vi "Database.vi"() -> ()   [LabVIEW 2016]
uses:
  Database.Data.ctl
  Database.Data.Sets.ctl
  Handler/Database.Handler.Data.Status.ctl
  Database.Action.ctl
  Tools/CitTemplate/citTemplate.errData.ctl
  Tools/EventLog/EventLog.EventSource.ctl
  Database.Global.vi
panel:
  out "error.action":string
  out "error":errorcluster
  out "_loop":i32(ring)=4
  out "action":T1=enum."--- DB ---"
  out "Data":T2
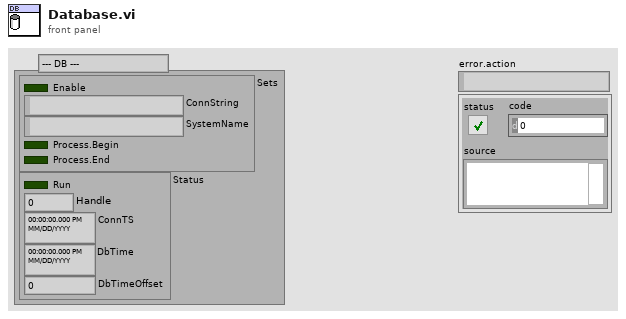
[diagram p1: front panel]
types:
  T1 = typedef "Database.Action.ctl" = enum32{"idle", "constructor", "destructor", "--- DB ---", "Setup", "Disconnect", "Connect", "GetAllStatuses"}
  T2 = typedef "Database.Data.ctl" = cluster{"Sets":T3, "Status":T4}
  T3 = typedef "Database.Data.Sets.ctl" = cluster{"Enable":bool, "ConnString":string, "SystemName":string, "Process.Begin":bool, "Process.End":bool}
  T4 = typedef "Database.Handler.Data.Status.ctl" = cluster{"Run":bool, "Handle":i32, "ConnTS":timestamp, "DbTime":timestamp, "DbTimeOffset":dbl}
  T5 = typedef "citTemplate.errData.ctl" = cluster{"ts":timestamp, "src":T6, "instance":i32, "action":string, "error":errorcluster, "unconfirmed":bool}
  T6 = typedef "EventLog.EventSource.ctl" = enum16{"All", "Gui", "Cache", "PLC1", "PLC2", "PLC3", "DB", "DB01", "DB02", "DB03", "DB04", "DB05", "DB06", "DB07", "DB08", "DB09", "DB10", "DB11", "DB12", "DB13", "DB14", "DB15", "DB16"}
  T7 = typedef "citTemplate.notifierHandle.ctl" = refnum<notifier>
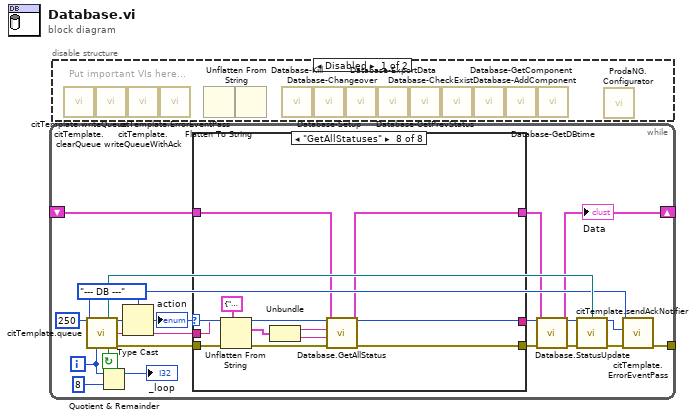
[diagram p0: block diagram]
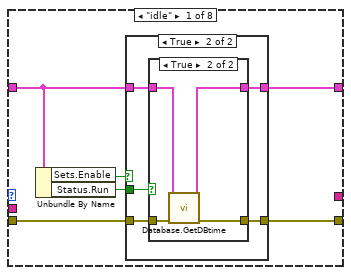
[diagram p3: hidden frame]
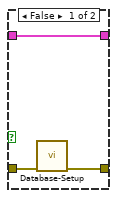
[diagram p5: hidden frame]
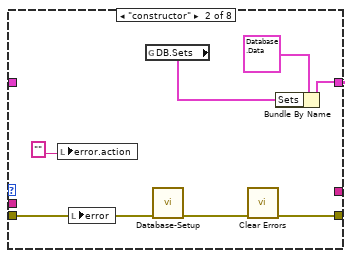
[diagram p6: hidden frame]
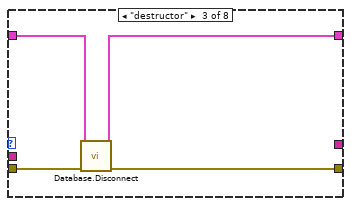
[diagram p7: hidden frame]
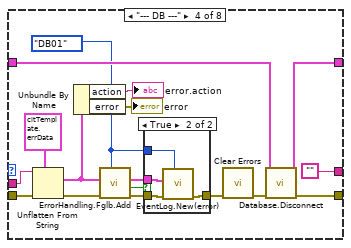
[diagram p8: hidden frame]
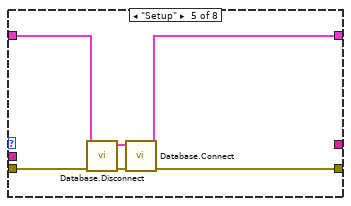
[diagram p10: hidden frame]
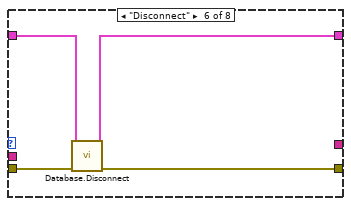
[diagram p11: hidden frame]
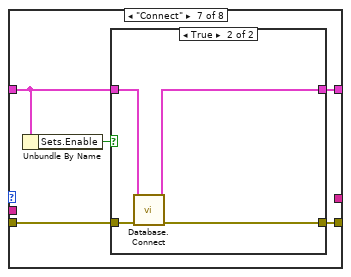
[diagram p12: hidden frame]
diagram:
  n1 = while {
    tunnel: [w12] -> _
    shift-right: [w1] -> _
    shift-left: _ -> [w5]
    i -> [w13]
    stop <- w15 continue-if-true
    w6 = Database.Action."--- DB ---" ("Action")
    n2 = call "citTemplate.queue.vi"("ms timeout (250 ms)"=250, "event enum"=w6, "iteration (-1)"=w13) -> ("notifierHandle out"=w7:T7, "event out"=w18:u32, "(flatten) data out"=w17:string, "continue"=w15:bool, "error out"=w16:errorcluster)  [unwired: 2 in, 6 out]
    n3 = Quotient & Remainder(x=w13, y=8) -> (x-y*floor(x/y)=→"_loop":i32)  [unwired: 1 out]
    n4 = Type Cast(type=w6, x=w18) -> (*(type *) &x=w11:T1)
    "action" <- w11
    n5 = case shown="\"GetAllStatuses\"" w11 {
      tunnel: w17 -> [_ _ _ w59 _ _ _ w100]
      tunnel: w16 -> [w24 w44 w47 w65 w76 w80 w85 w101]
      tunnel: [w22 w43 w46 w61 w72 w78 w84 w96] -> w4
      tunnel: [w20 w40 w48 w62 w71 w77 w83 w94] -> w2
      tunnel: w5 -> [w21 _ w49 w63 w75 w79 w82 w95]
      tunnel: [_ _ _ "" _ _ _ _] -> w8
      frame "idle" {
        n6 = Unbundle By Name(w21) -> ("Sets.Enable"=w19:bool, "Status.Run"=w23:bool)
        n7 = case shown="True" w19 {
          tunnel: w24 -> [w25 w31]
          tunnel: w23 -> [_ w30]
          tunnel: [w25 w29] -> w22
          tunnel: w21 -> [w26 w28]
          tunnel: [w26 w27] -> w20
          frame False {
          }
          frame True {
            n8 = case shown="True" w30 {
              tunnel: w31 -> [w33 w36]
              tunnel: [w32 w35] -> w29
              tunnel: w28 -> [w34 w38]
              tunnel: [w34 w37] -> w27
              frame False {
                n9 = call "Database-Setup.vi"("error in"=w33) -> ("error out"=w32:errorcluster)  [unwired: 10 in]
              }
              frame True {
                n10 = call "Database.GetDBtime.vi"("error in (no error)"=w36, "Data in"=w38) -> ("error out"=w35:errorcluster, "Data out"=w37:T2)  [unwired: 8 in]
              }
            }
          }
        }
      }
      frame "constructor" {
        n11 = local write "error.action"("" ("error.action")) -> ()
        n12 = local write "error"(w44) -> ()
        n13 = global read "Database.Global.vi" "DB.Sets"() -> (w39:T3)
        n14 = call "Database-Setup.vi"("error in"=w44) -> ("error out"=w42:errorcluster)  [unwired: 10 in]
        n15 = call <vilib>:"Clear Errors.vi"("error in (no error)"=w42) -> ("error out"=w43:errorcluster)  [unwired: 5 in, 1 out]
        n16 = Bundle By Name(cluster=T2 {"Sets"={"Enable"=FALSE, "ConnString"="", "SystemName"="", "Process.Begin"=FALSE, "Process.End"=FALSE}, "Status"={"Run"=FALSE, "Handle"=0, "ConnTS"=timestamp(0 s since 1904-01-01), "DbTime"=timestamp(0 s since 1904-01-01), "DbTimeOffset"=0.0}} ("Data out"), "Sets"=w39) -> (w40:T2)
      }
      frame "destructor" {
        n17 = call "Database.Disconnect.vi"("error in (no error)"=w47, "Data in"=w49) -> ("error out"=w46:errorcluster, "Data out"=w48:T2)  [unwired: 8 in]
      }
      frame "--- DB ---" {
        w50 = EventLog.EventSource."DB01" ("Event source")
        n18 = Unflatten From String(type=T5 {"ts"=timestamp(0 s since 1904-01-01), "src"=enum."All", "instance"=0, "action"="", "error"={"status"=FALSE, "code"=0, "source"=""}, "unconfirmed"=FALSE} ("ErrData"), binary string=w59, error in (no error)=w65) -> (value=w52:T5, error out=w55:errorcluster)  [unwired: 3 out]
        n19 = Unbundle By Name(w52) -> ("action"=→"error.action":string, "error"=→"error":errorcluster)
        n20 = call "ErrorHandling.Fglb.Add.vi"("Event source"=w50, "error in (no error)"=w55, "Error in"=w52) -> ("error out"=w57:errorcluster, "changed?"=w56:bool)  [unwired: 7 in]
        n21 = case shown="True" w56 {
          tunnel: [w66 w70] -> w54
          tunnel: w52 -> [_ w69]
          tunnel: w57 -> [w66 w68]
          tunnel: w50 -> [_ w67]
          frame False {
          }
          frame True {
            n22 = call "EventLog.New(error).vi"("Source (All)"=w67, "error in"=w68, "ErrData"=w69) -> ("error out"=w70:errorcluster)  [unwired: 8 in]
          }
        }
        n23 = call <vilib>:"Clear Errors.vi"("error in (no error)"=w54) -> ("error out"=w60:errorcluster)  [unwired: 5 in, 1 out]
        n24 = call "Database.Disconnect.vi"("error in (no error)"=w60, "Data in"=w63) -> ("error out"=w61:errorcluster, "Data out"=w62:T2)  [unwired: 8 in]
      }
      frame "Setup" {
        n25 = call "Database.Disconnect.vi"("error in (no error)"=w76, "Data in"=w75) -> ("error out"=w73:errorcluster, "Data out"=w74:T2)  [unwired: 8 in]
        n26 = call "Database.Connect.vi"("error in"=w73, "Data in"=w74) -> ("error out"=w72:errorcluster, "Data out"=w71:T2)  [unwired: 8 in]
      }
      frame "Disconnect" {
        n27 = call "Database.Disconnect.vi"("error in (no error)"=w80, "Data in"=w79) -> ("error out"=w78:errorcluster, "Data out"=w77:T2)  [unwired: 8 in]
      }
      frame "Connect" {
        n28 = Unbundle By Name(w82) -> ("Sets.Enable"=w81:bool)
        n29 = case shown="True" w81 {
          tunnel: w85 -> [w87 w91]
          tunnel: [w87 w89] -> w84
          tunnel: [w86 w88] -> w83
          tunnel: w82 -> [w86 w90]
          frame False {
          }
          frame True {
            n30 = call "Database.Connect.vi"("error in"=w91, "Data in"=w90) -> ("error out"=w89:errorcluster, "Data out"=w88:T2)  [unwired: 8 in]
          }
        }
      }
      frame "GetAllStatuses" {
        n31 = Unflatten From String(type=cluster{"Ref":string, "Serial":string} {"Ref"="", "Serial"=""} ("cluster"), binary string=w100, error in (no error)=w101) -> (value=w98:cluster{"Ref":string, "Serial":string}, error out=w97:errorcluster)  [unwired: 2 in, 1 out]
        n32 = Unbundle(w98) -> ("Ref"=w93:string, "Serial"=w92:string)
        n33 = call "Database.GetAllStatus.vi"("error in"=w97, "Serial"=w92, "Variant"=w93, "Data in"=w95) -> ("error out"=w96:errorcluster, "Data out"=w94:T2)  [unwired: 6 in]
      }
    }
    n34 = call "Database.StatusUpdate.vi"("error in (no error)"=w4, "Data in"=w2) -> ("error out"=w3:errorcluster, "Data out"=w1:T2)  [unwired: 8 in]
    "Data" <- w1
    n35 = call "citTemplate.sendAckNotifier.vi"("notification data"=w8, "notifierHandle in"=w7, "error in"=w3) -> ()  [unwired: 13 in]
    n36 = call "citTemplate.ErrorEventPass.vi"("error in"=w3, "action of error"=w11, "event in"=w6) -> ("error out"=w12:errorcluster)  [unwired: 2 in, 6 out]
  }
  n37 = disable-structure shown="Disabled" {
    frame Disabled {
      # "Put important VIs here..."
      n38 = call "citTemplate.clearQueue.vi"() -> ()  [unwired: 14 in, 2 out]
      n39 = call "citTemplate.writeQueue.vi"() -> ()  [unwired: 15 in, 1 out]
      n40 = call "citTemplate.writeQueueWithAck.vi"() -> ()  [unwired: 13 in, 3 out]
      n41 = call "citTemplate.ErrorEventPass.vi"() -> ()  [unwired: 11 in, 1 out]
      n42 = Flatten To String() -> ()  [unwired: 4 in, 3 out]
      n43 = Unflatten From String() -> ()  [unwired: 5 in, 3 out]
      n44 = call "Database-Kill.vi"() -> ()  [unwired: 11 in, 1 out]
      n45 = call "Database-Setup.vi"() -> ()  [unwired: 11 in, 1 out]
      n46 = call "Database-Changeover.vi"() -> ()  [unwired: 10 in, 2 out]
      n47 = call "Database-ExportData.vi"() -> ()  [unwired: 9 in, 3 out]
      n48 = call "Database-GetPrevStatus.vi"() -> ()  [unwired: 10 in, 2 out]
      n49 = call "Database-CheckExist.vi"() -> ()  [unwired: 11 in, 1 out]
      n50 = call "Database-AddComponent.vi"() -> ()  [unwired: 11 in, 1 out]
      n51 = call "Database-GetComponent.vi"() -> ()  [unwired: 9 in, 3 out]
      n52 = call "Database-GetDBtime.vi"() -> ()  [unwired: 1 in, 1 out]
      n53 = call "ProdaNG.Configurator.vi"() -> ()  [unwired: 12 in]
    }
    frame Enabled {
    }
  }
